vi "Result.vi"(8 "error in (no error)":errorcluster, 10 "Result":T1={"Name"="", "Message"="", "Description"="", "Status"=enum."Passed", "Result Type"=enum."Case", "Execution Time"=0.0}, 11 "Icon Decorator V2 in":refnum<class "Icon Decorator V2.lvclass">) -> (0 "error out":errorcluster, 3 "Icon Decorator V2 out":refnum<class "Icon Decorator V2.lvclass">)   [LabVIEW 2020, in "Icon Decorator V2.lvclass"]
uses:
  Icon Decorator V2.lvclass
  Result/Result.ctl
  Result/Status.ctl
  Result/Type.ctl
  Result/Result.lvlib
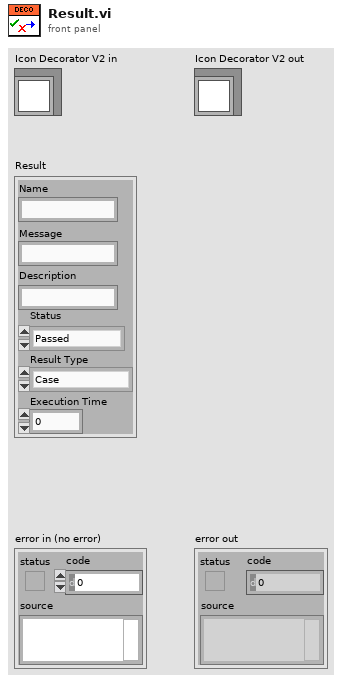
[diagram p1: front panel]
types:
  T1 = typedef "Result.lvlib/Result.ctl" = cluster{"Name":string, "Message":string, "Description":string, "Status":T2, "Result Type":T3, "Execution Time":dbl}
  T2 = typedef "Result.lvlib/Status.ctl" = enum16{"None", "Passed", "Failed", "Error", "Skipped", "Setup Error", "Broken", "Teardown Error"}
  T3 = typedef "Result.lvlib/Type.ctl" = enum16{"Method", "Case", "Suite", "Pass", "Fail", "Skip", "Pass if", "Fail if", "Pass if Error", "Fail if Error", "Pass if Equal", "Fail if Equal"}
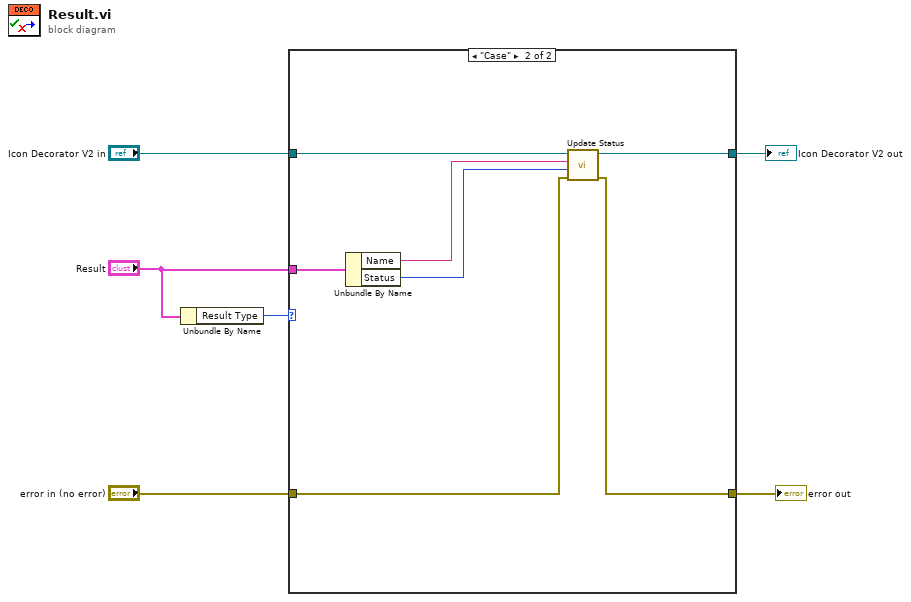
[diagram p0: block diagram]
diagram:
  n1 = Unbundle By Name("Result") -> ("Result Type"=w6:T3)
  n2 = case shown="\"Case\"" w6 {
    tunnel: "Icon Decorator V2 in" -> [w8 w12]
    tunnel: [w8 w13] -> w4
    tunnel: "error in (no error)" -> [w7 w10]
    tunnel: "Result" -> [_ w15]
    tunnel: [w7 w9] -> w1
    frame Default {
    }
    frame "Case" {
      n3 = Unbundle By Name(w15) -> ("Name"=w14:string, "Status"=w11:T2)
      n4 = call "Update Status.vi"("error in (no error)"=w10, "Status"=w11, "Case"=w14, "Icon Decorator V2 In"=w12) -> ("error out"=w9:errorcluster, "Icon Decorator V2 Out"=w13:refnum<class "Icon Decorator V2.lvclass">)  [unwired: 6 in]
    }
  }
  "error out" <- w1
  "Icon Decorator V2 out" <- w4
